vi "Write_data_to_text_file.vi"(11 ".CSV? (F=.txt)":bool=TRUE) -> ()   [LabVIEW 2017, in "labview-standard-library.lvlib"]
doc: "Gets binary file data and turns it into human readable plain ASCII text or .CSV spreadsheet file."
uses:
  labview-standard-library.lvlib
  Event_log_binary_data.ctl
  Time&Event_cluster.ctl
  <vilib>/Utility/file.llb/Write Delimited Spreadsheet (string).vi
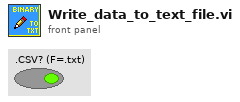
[diagram p1: front panel]
types:
  T1 = typedef "labview-standard-library.lvlib/Event_log_binary_data.ctl" = cluster{"path":path, "Time/Event":T2[]}
  T2 = typedef "labview-standard-library.lvlib/Time&Event_cluster.ctl" = cluster{"Time in seconds":dbl, "Event text":string}
  T3 = enum16{"open", "replace", "create", "open or create", "replace or create", "replace or create with confirmation"}
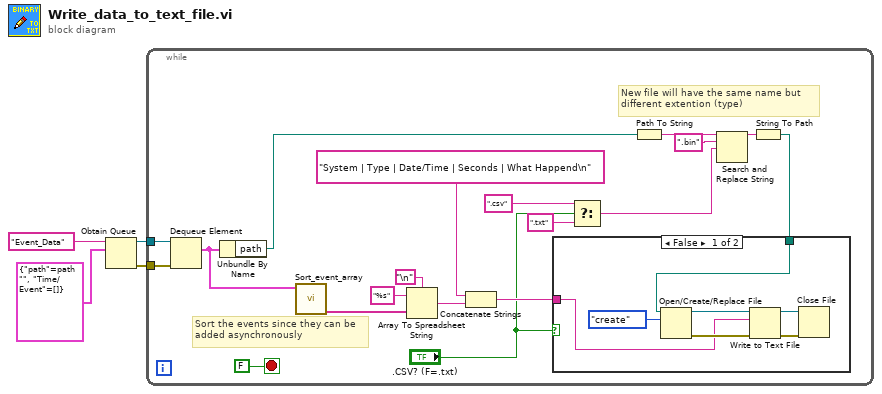
[diagram p0: block diagram]
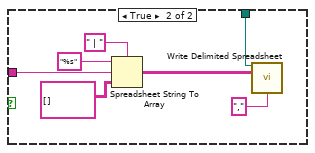
[diagram p2: hidden frame]
diagram:
  n1 = Obtain Queue(name (unnamed)="Event_Data", element data type=T1 {"path"=path "", "Time/Event"=[]} ("Cluster")) -> (queue out=w2:refnum<queue>, error out=w1:errorcluster)  [unwired: 3 in, 1 out]
  n2 = while {
    tunnel: w2 -> [w13]
    tunnel: w1 -> [w14]
    stop <- FALSE stop-if-true
    # "Sort the events since they can be\nadded asynchronously"
    # "New file will have the same name but\ndifferent extention (type)"
    n3 = Dequeue Element(queue=w13, error in (no error)=w14) -> (element=w5:T1)  [unwired: 1 in, 3 out]
    n4 = Unbundle By Name(w5) -> ("path"=w12:path)
    n5 = call "Sort_event_array.vi"("Data cluster in"=w5) -> ("sorted event array"=w6:string[])  [unwired: 10 in]
    n6 = Array To Spreadsheet String(delimiter (Tab)="\n", array=w6, 3:"%s" ("format string")) -> (spreadsheet string=w18:string)
    n7 = Concatenate Strings("System | Type | Date/Time | Seconds | What Happend\n", w18) -> (w17:string)
    n8 = Select(t=".csv" ("replace string (\"\")"), s=".CSV? (F=.txt)", f=".txt") -> (s? t:f=w9:string)
    n9 = Path To String(path=w12) -> (string=w20:string)
    n10 = Search and Replace String(input string=w20, search string=".bin", replace string=w9) -> (result string=w22:string)  [unwired: 5 in, 3 out]
    n11 = String To Path(string=w22) -> (path=w23:path)
    n12 = case shown="False" ".CSV? (F=.txt)" {
      tunnel: w23 -> [w25 w36]
      tunnel: w17 -> [w24 w35]
      frame False {
        n13 = Open/Create/Replace File(file path (use dialog)=w25, operation (0:open)=T3."create") -> (refnum out=w30:refnum<file>, error out=w28:errorcluster)  [unwired: 4 in, 1 out]
        n14 = Write to Text File(file (use dialog)=w30, text=w24, error in=w28) -> (refnum out=w26:refnum<file>, error out=w27:errorcluster)  [unwired: 1 in, 1 out]
        n15 = Close File(refnum=w26, error in=w27) -> ()  [unwired: 2 out]
      }
      frame True {
        n16 = Spreadsheet String To Array(delimiter (Tab)=" | ", format string="%s", spreadsheet string=w35, array type (2D Dbl)=string[][] []) -> (array=w31:string[][])
        n17 = call-poly <vilib>:"Write Delimited Spreadsheet.vi"("file path (dialog if empty)"=w36, "2D data"=w31, "delimiter (\\t)"="," ("delimiter (\\t)")) -> ()  [unwired: 11 in, 2 out]
      }
    }
  }
